vi "loadDataNodeEnd.vi"(8 "error in (no error)":errorcluster, 10 "XML Refnum in":refnum<file>, 11 "DMA_Read in":refnum<class "DMA_Read.lvclass">) -> (0 "error out":errorcluster, 2 "XML Refnum out":refnum<file>, 3 "DMA_Read out":refnum<class "DMA_Read.lvclass">)   [LabVIEW 2013, in "DMA_Read.lvclass"]
doc: "Part of the file loading process. Occurs at the end of a node being loaded. Includes checking the end of the tag which has the format </tag>."
uses:
  DMA_Read.lvclass
  xCE/xceDataNode/xceDataNode.lvclass
  XML Parser/XML Parser.lvclass
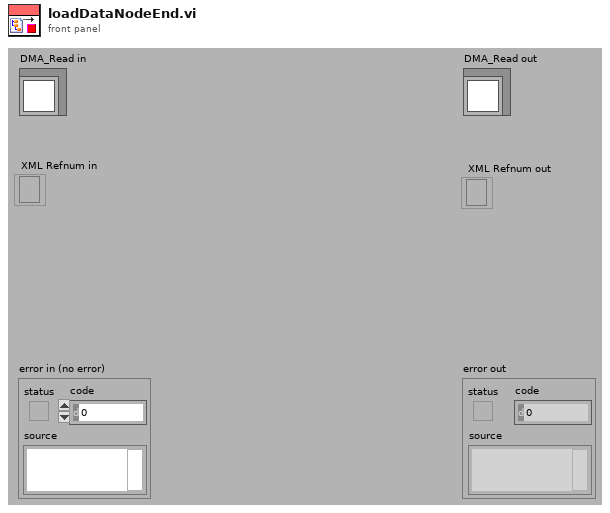
[diagram p1: front panel]
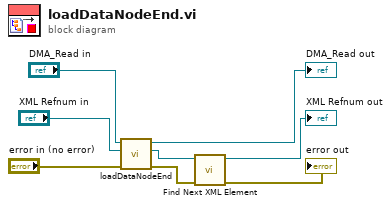
[diagram p0: block diagram]
diagram:
  n1 = call-parent "loadDataNodeEnd.vi"("error in (no error)"="error in (no error)", "XML Refnum in"="XML Refnum in", "xceDataNode in"="DMA_Read in") -> ("error out"=w3:errorcluster, "XML Refnum out"=w4:refnum<file>, "xceDataNode out"=→"DMA_Read out":refnum<class "DMA_Read.lvclass">)  [unwired: 6 in]
  n2 = call "Find Next XML Element.vi"("error in (no error)"=w3, "XML Fine In"=w4) -> ("error out"=→"error out":errorcluster, "XML Fine Out"=→"XML Refnum out":refnum<file>)  [unwired: 7 in, 1 out]
